vi "Const - Cannel Names.vi"() -> (0 "Channel Name":string[](array[string])=["Уровень  масла", "Уровень  масла", "Температура масла", "Температура масла", "давление после насоса ВД", "Давление в образце", "Давление в камере", "Давление  в  линии подачи воздуха в  блок ППВ", "Давление  в  линии подачи воздуха после блока ППВ", "Датчик давления в линии измерения утечек"])   [LabVIEW 2019]
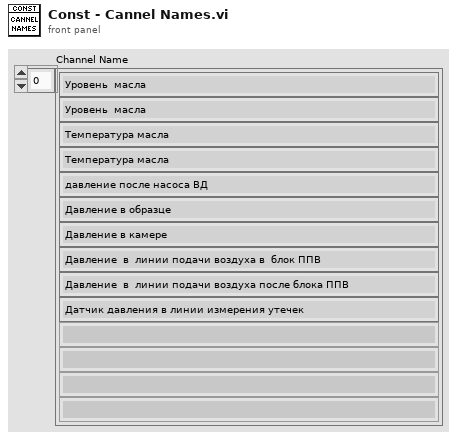
[diagram p1: front panel]
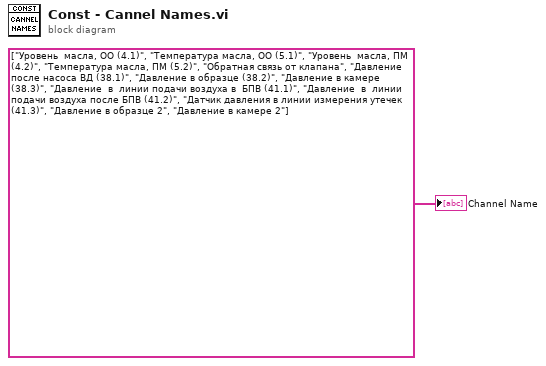
[diagram p0: block diagram]
diagram:
  "Channel Name" <- string[] ["Уровень  масла, ОО (4.1)", "Температура масла, ОО (5.1)", "Уровень  масла, ПМ (4.2)", "Температура масла, ПМ (5.2)", "Обратная связь от клапана", "Давление после насоса ВД (38.1)", "Давление в образце (38.2)", "Давление в камере (38.3)", "Давление  в  линии подачи воздуха в  БПВ (41.1)", "Давление  в  линии подачи воздуха после БПВ (41.2)", "Датчик давления в линии измерения утечек (41.3)", "Давление в образце 2", "Давление в камере 2"]
